vi "StyledText.Example.vi"() -> ()   [LabVIEW 2010]
doc: "<i>Copyright (c) 2018, Martin Weiss\nAll rights reserved.</i>\n\nRedistribution and use in source and binary forms, with or without modification, are permitted provided that the following conditions are met:\n\n1. Redistributions of source code must retain the above copyright notice, this list of conditions and the following disclaimer.\n\n2. Redistributions in binary form must reproduce the above copyright notice, this list of conditions and the following disclaimer in the documentation and/or other materials provided with the distribution.\n\nTHIS SOFTWARE IS PROVIDED BY THE COPYRIGHT HOLDERS AND CONTRIBUTORS \"AS IS\" AND ANY EXPRESS OR IMPLIED WARRANTIES, INCLUDING, BUT NOT LIMITED TO, THE IMPLIED WARRANTIES OF MERCHANTABILITY AND FITNESS FOR A PARTICULAR PURPOSE ARE DISCLAIMED. IN NO EVENT SHALL THE COPYRIGHT HOLDER OR CONTRIBUTORS BE LIABLE FOR ANY DIRECT, INDIRECT, INCIDENTAL, SPECIAL, EXEMPLARY, OR CONSEQUENTIAL DAMAGES (INCLUDING, BUT NOT LIMITED TO, PROCUREMENT OF SUBSTITUTE GOODS OR SERVICES; LOSS OF USE, DATA, OR PROFITS; OR BUSINESS INTERRUPTION) HOWEVER CAUSED AND ON ANY THEORY OF LIABILITY, WHETHER IN CONTRACT, STRICT LIABILITY, OR TORT (INCLUDING NEGLIGENCE OR OTHERWISE) ARISING IN ANY WAY OUT OF THE USE OF THIS SOFTWARE, EVEN IF ADVISED OF THE POSSIBILITY OF SUCH DAMAGE."
uses:
  StyledText/StyledText.lvlib
  Licenses.lvlib
panel:
  in  "String":string="This is <i><b>styled</b></i> text. You can change <font color=\"#ff0000\">c</font><font color=\"#00ff00\">o</font><font color=\"#0000ff\">l</font><font color=\"#000000\">o</font><font color=\"#ffffff\">r</font>, <font size=\"30\">size</font>, the <font face=\"Courier\">font</font> or its parameters <b>bold</b>, <i>italic</i>, <s>strikeout</s> or <u>underline</u>. Note that the characters &lt; &gt; and &amp; must be quoted as in XML."
  out "StyledText":string
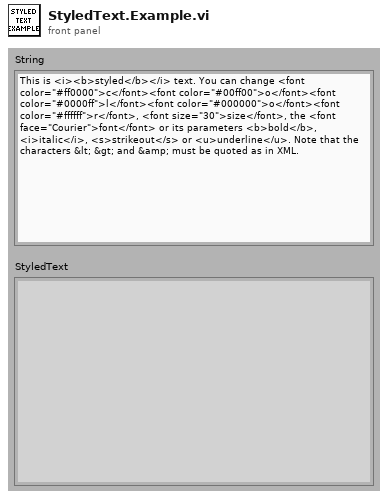
[diagram p1: front panel]
types:
  T1 = enum32{"invalid app kind", "Development System", "Run Time System", "Student Edition", "Embedded LabVIEW", "Evaluation", "Custom"}
  T2 = typedef "FileVersionInformation.ctl" = cluster{"FileVersion":string, "ProductName":string, "InternalName":string, "CompanyName":string, "LegalCopyright":string, "FileDescription":string}
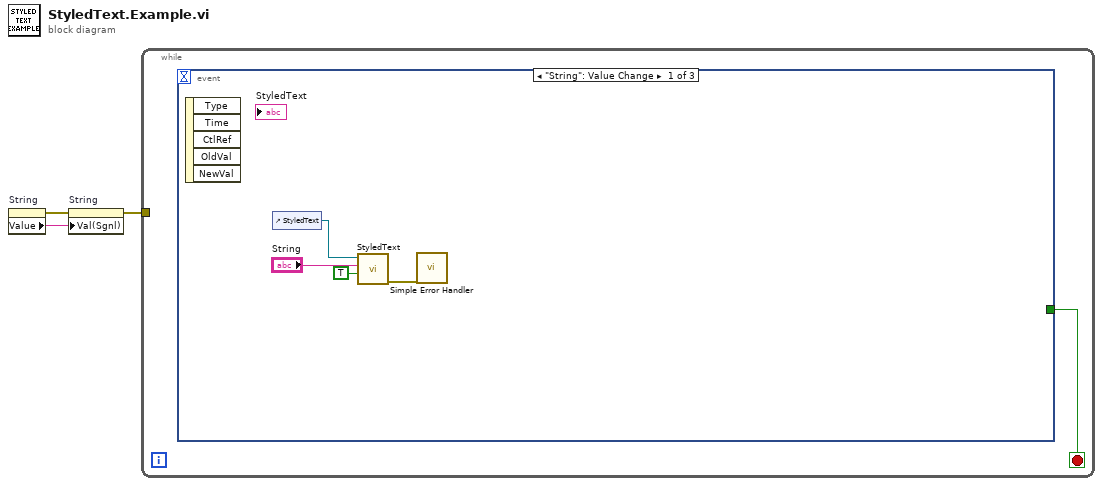
[diagram p0: block diagram]
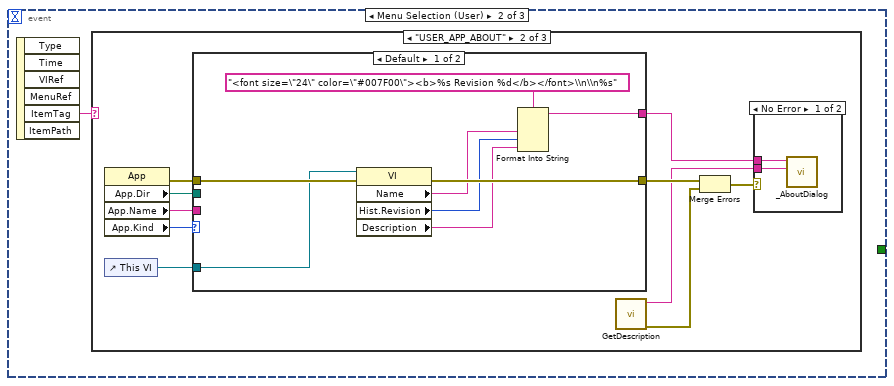
[diagram p2: hidden frame]
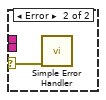
[diagram p4: hidden frame]
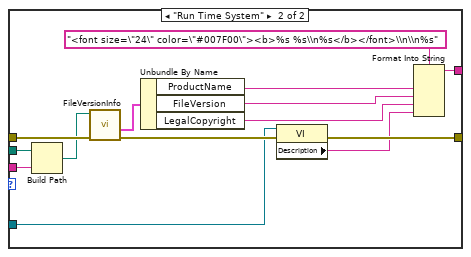
[diagram p5: hidden frame]
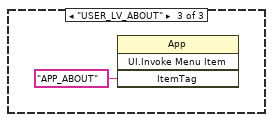
[diagram p6: hidden frame]
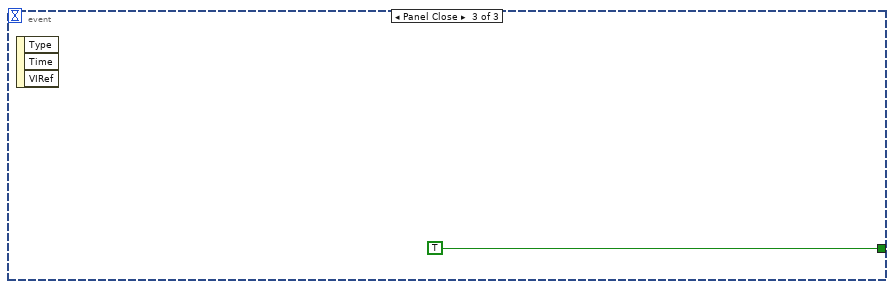
[diagram p7: hidden frame]
diagram:
  n1 = property on="String" class="Str"() -> (error out=w3:errorcluster, "Value"=w2:string)  [unwired: 2 in, 1 out]
  n2 = property on="String" class="Str"(error in=w3, "Val(Sgnl)"=w2) -> (error out=w1:errorcluster)  [unwired: 1 in, 1 out]
  n3 = while {
    tunnel: w1 -> [_]
    stop <- w4 stop-if-true
    n4 = event shown="[0] \"String\": Value Change" {
      selector: _ -> [_ _ _]
      dyn-events: _ -> [_ _ _]
      timeout: _ -> [_ _ _]
      tunnel: [_ _ TRUE] -> w4
      event "String": Value Change {
        n5 = event-data() -> ()  [unwired: 1 in, 5 out]
        n6 = control-ref of="StyledText"() -> (w6:refnum<vi>)
        n7 = call "StyledText.vi"("deferPanelUpdates in"=TRUE, "text in"="String", "StringControl"=w6) -> ("error out"=w7:errorcluster)  [unwired: 8 in]
        n8 = call <vilib>:"Simple Error Handler.vi"("error in (no error)"=w7) -> ()  [unwired: 4 in, 5 out]
      }
      event Menu Selection (User) {
        n9 = event-data() -> ("ItemTag"=w9:string)  [unwired: 1 in, 5 out]
        n10 = case shown="\"USER_APP_ABOUT\"" w9 {
          frame Default {
          }
          frame "USER_APP_ABOUT" {
            n11 = property class="App"() -> (error out=w17:errorcluster, "App.Dir"=w18:path, "App.Name"=w19:string, "App.Kind"=w16:T1)  [unwired: 2 in, 1 out]
            n12 = control-ref of="This VI"() -> (w15:refnum<vi>)
            n13 = case shown="Default" w16 {
              tunnel: w19 -> [_ w44]
              tunnel: w18 -> [_ w43]
              tunnel: w17 -> [w30 w42]
              tunnel: [w29 w33] -> w14
              tunnel: [w27 w34] -> w11
              tunnel: w15 -> [w23 w31]
              frame Default {
                n14 = property class="VI"(reference=w23, error in=w30) -> (error out=w29:errorcluster, "Name"=w26:string, "Hist.Revision"=w25:u32, "Description"=w24:string)  [unwired: 1 out]
                n15 = Format Into String(format string="<font size=\"24\" color=\"#007F00\"><b>%s Revision %d</b></font>\\n\\n%s", w26, w25, w24) -> (resulting string=w27:string)  [unwired: 2 in, 1 out]
              }
              frame "Run Time System" {
                n16 = Build Path(base path=w43, name or relative path=w44) -> (appended path=w41:path)
                n17 = call <vilib>:"FileVersionInfo.vi"("error in (no error)"=w42, "Application Path in"=w41) -> ("error out"=w35:errorcluster, "FileVersionInfo Out"=w40:T2)  [unwired: 6 in, 2 out]
                n18 = Unbundle By Name(w40) -> ("ProductName"=w39:string, "FileVersion"=w38:string, "LegalCopyright"=w37:string)
                n19 = property class="VI"(reference=w31, error in=w35) -> (error out=w33:errorcluster, "Description"=w32:string)  [unwired: 1 out]
                n20 = Format Into String(format string="<font size=\"24\" color=\"#007F00\"><b>%s %s\\n%s</b></font>\\n\\n%s", w39, w38, w37, w32) -> (resulting string=w34:string)  [unwired: 2 in, 1 out]
              }
            }
            n21 = call "GetDescription.vi"() -> ("error out"=w13:errorcluster, "text out"=w10:string)  [unwired: 10 in]
            n22 = Merge Errors(w14, w13) -> (w12:errorcluster)
            n23 = case shown="No Error" w12 {
              selector: w12 -> [_ w22]
              tunnel: w11 -> [w21 _]
              tunnel: w10 -> [w20 _]
              frame No Error {
                n24 = call "_AboutDialog.vi"("libsAndLicenseInfo in"=w20, "applicationInfo in"=w21) -> ()  [unwired: 10 in]
              }
              frame Error {
                n25 = call <vilib>:"Simple Error Handler.vi"("error in (no error)"=w22) -> ()  [unwired: 4 in, 5 out]
              }
            }
          }
          frame "USER_LV_ABOUT" {
            n26 = invoke class="App" method="UI.Invoke Menu Item"("ItemTag"="APP_ABOUT" ("Menu Item Tag")) -> ()  [unwired: 3 in, 4 out]
          }
        }
      }
      event Panel Close {
        n27 = event-data() -> ()  [unwired: 1 in, 3 out]
      }
    }
  }
